vi "Errorcalculator.vi"() -> ()   [LabVIEW 2020]
uses:
  <vilib>/Analysis/NI_AALBase.lvlib
  <vilib>/Analysis/NI_AALPro.lvlib
panel:
  out "mse":dbl format="%0.2f"
  out "variance":dbl format="%0.2f"
  out "standard deviation":dbl format="%0.2f"
  out "mean":dbl format="%0.2f"
  out "output array":dbl[](array[numeric])
  out "subarray":dbl[][](array[numeric])
  out "x > y?":bool
  out "Array 2":dbl[][](array[numeric])
  out "initialized array":dbl[][](array[numeric])
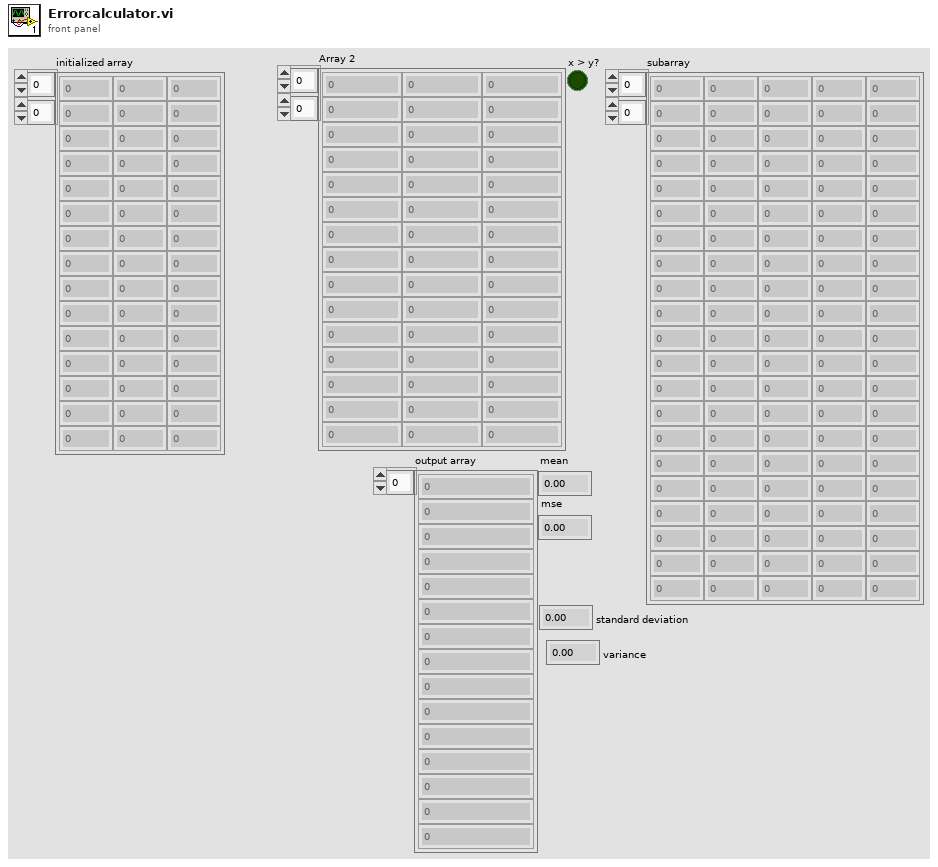
[diagram p1: front panel]
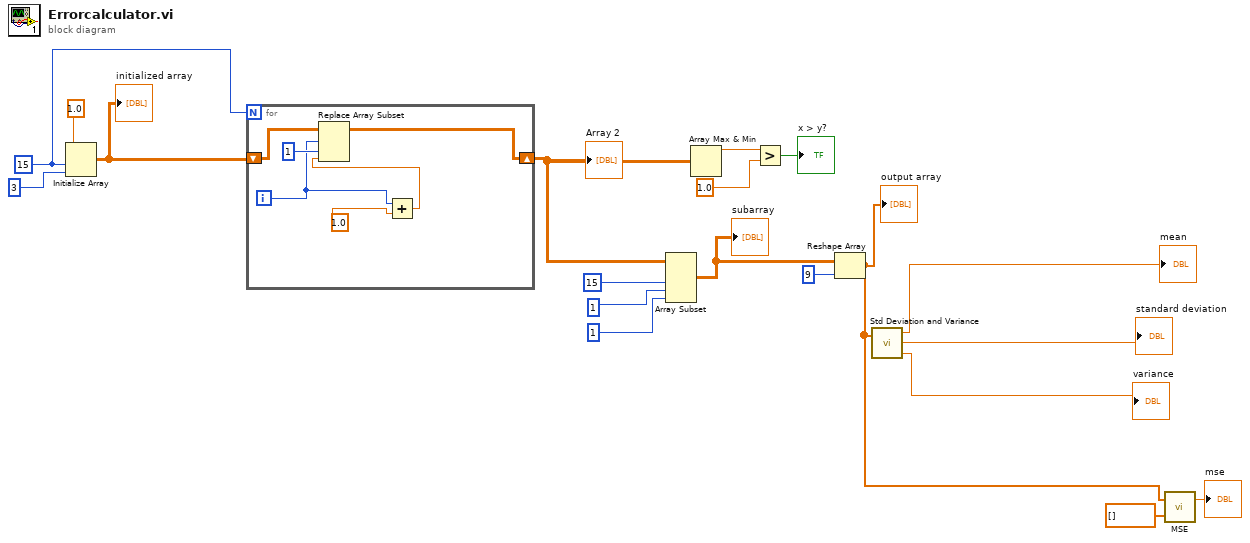
[diagram p0: block diagram]
diagram:
  w16 = 15 ("dimension size")
  n1 = Initialize Array(1.0 ("element"), w16, 3 ("dimension size")) -> (w17:dbl[][])
  "initialized array" <- w17
  n2 = for {
    N: w16 -> [_]
    shift-right: [w24] -> w12
    shift-left: w17 -> [w25]
    i -> [w21]
    n3 = Add(x=w21, y=1.0 ("new element/subarray")) -> (x+y=w20:dbl)
    n4 = Replace Array Subset(array=w25, new element=w20, index (row)=w21, index (col)=1 ("disabled index (col)")) -> (w24:dbl[][])
  }
  "Array 2" <- w12
  n5 = Array Subset(array=w12, length (row)=15 ("length"), index (col)=1 ("index"), length (col)=1 ("length")) -> (w8:dbl[][])  [unwired: 1 in]
  "subarray" <- w8
  n6 = Array Max & Min(array=w12) -> (max value=w15:dbl)  [unwired: 3 out]
  n7 = Greater?(x=w15, y=1.0) -> (0:→"x > y?":bool)
  n8 = Reshape Array(w8, 9 ("dimension size")) -> (w3:dbl[])
  "output array" <- w3
  n9 = call <vilib>:"Std Deviation and Variance.vi"("X"=w3) -> ("mean"=→"mean":dbl, "standard deviation"=→"standard deviation":dbl, "variance"=→"variance":dbl)  [unwired: 1 in]
  n10 = call <vilib>:"MSE.vi"("X Values"=dbl[] [], "Y Values"=w3) -> ("mse"=→"mse":dbl)  [unwired: 1 out]
